vi "_PC_Pub_DBL2FiniteDigString.vi"(9 "Digit":i32, 10 "DBL in":dbl) -> (2 "String out":string)   [LabVIEW 2018]
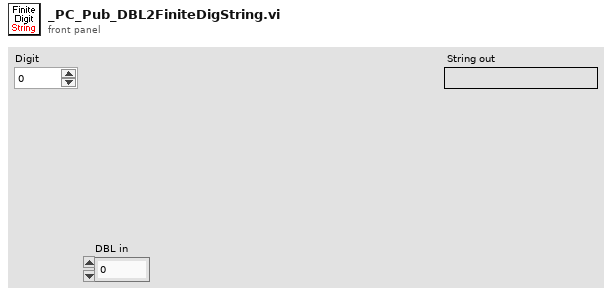
[diagram p1: front panel]
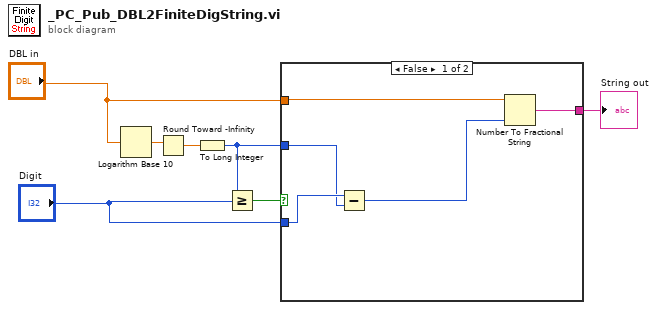
[diagram p0: block diagram]
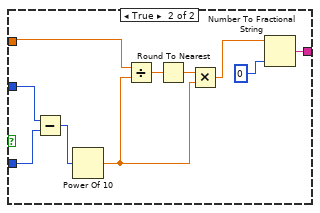
[diagram p2: hidden frame]
diagram:
  n1 = Logarithm Base 10(1:"DBL in") -> (0:w6:dbl)
  n2 = Round Toward -Infinity(1:w6) -> (0:w4:dbl)
  n3 = To Long Integer(number=w4) -> (32bit integer=w5:i32)
  n4 = Greater Or Equal?(x=w5, y="Digit") -> (x >= y?=w7:bool)
  n5 = case shown="False" w7 {
    tunnel: "DBL in" -> [w12 w20]
    tunnel: [w8 w21] -> w3
    tunnel: w5 -> [w10 w15]
    tunnel: "Digit" -> [w11 w14]
    frame False {
      n6 = Subtract(x=w11, y=w10) -> (x-y=w9:i32)
      n7 = Number To Fractional String(number=w12, precision (6)=w9) -> (F-format string=w8:string)  [unwired: 2 in]
    }
    frame True {
      n8 = Subtract(x=w15, y=w14) -> (x-y=w13:i32)
      n9 = Power Of 10(x=w13) -> (10^x=w17:dbl)
      n10 = Divide(x=w20, y=w17) -> (x/y=w19:dbl)
      n11 = Round To Nearest(number=w19) -> (nearest integer value=w18:dbl)
      n12 = Multiply(x=w18, y=w17) -> (x*y=w16:dbl)
      n13 = Number To Fractional String(number=w16, precision (6)=i16 0) -> (F-format string=w21:string)  [unwired: 2 in]
    }
  }
  "String out" <- w3
